vi "Cycle Write.vi"(4 "error in (no error)":errorcluster, 5 "Value":dbl=1.0, 6 "Container State":T2, 7 "Display State In":T1={"cycle"=1.0, "timing vi"=refnum, "NISAST Event.lvclass"=refnum}) -> (0 "error out":errorcluster, 3 "Display State Out":T1={"cycle"=1.0, "timing vi"=refnum, "NISAST Event.lvclass"=refnum})   [LabVIEW 2010, in "Twinkle Button.xctl"]
doc: "本VI是为《我和LabVIEW》一书编写的示例。\n关于本书的介绍请参考网页：\nhttp://ruanqizhen.spaces.live.com/blog/cns!5852D4F797C53FB6!4310.entry"
uses:
  Twinkle Button.xctl
  <vilib>/_xctls/Container State.ctl
  State.ctl
  C:/Program Files/National Instruments/LabVIEW 2010/resource/importtools/Common/Event/NISAST Event.lvclass
  <vilib>/_xctls/XControlSupport.lvlib
panel:
  # "Replace the Value Control below with a Control of desired type.\nDo not remove this Control or the others from the connector pane.\nDo not change the connector pane pattern.\nThe Value control should always be the third terminal from top on the input side in the connector pane."
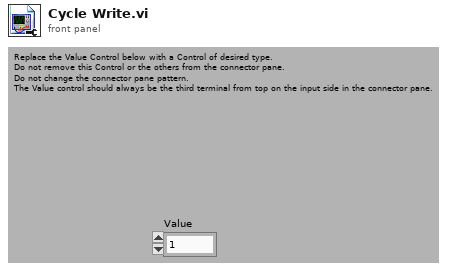
[diagram p1: front panel]
types:
  T1 = typedef "Twinkle Button.xctl/State.ctl" = cluster{"cycle":dbl, "timing vi":refnum<vi>, "NISAST Event.lvclass":refnum<class "NISAST Event.lvclass">}
  T2 = typedef "XControlSupport.lvlib/Container State.ctl" = cluster{"Indicator?":bool, "Run Mode?":bool, " Refnum":refnum<vi>}
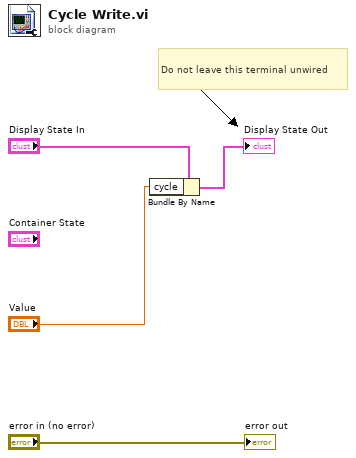
[diagram p0: block diagram]
diagram:
  # "Do not leave this terminal unwired"
  n1 = Bundle By Name(cluster="Display State In", "cycle"="Value") -> (→"Display State Out":T1)
  "error out" <- "error in (no error)"
